vi "Lire Dividend.vi"(8 "error in (no error)":errorcluster caption="entrée d'erreur (pas d'erreur)", 11 "Share en entrée":refnum<class "Stock.lvclass">) -> (0 "error out":errorcluster caption="sortie d'erreur", 2 "Dividend":dbl, 3 "Share en sortie":refnum<class "Stock.lvclass">)   [LabVIEW 2012, in "Stock.lvclass"]
uses:
  Stock.lvclass
  Stock.lvclass/Stock.ctl
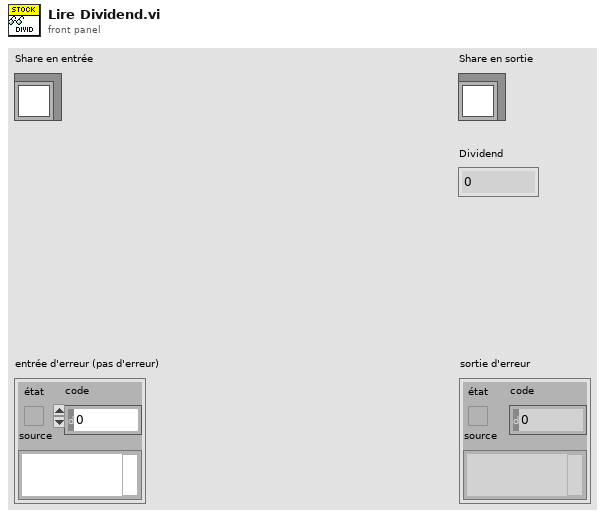
[diagram p1: front panel]
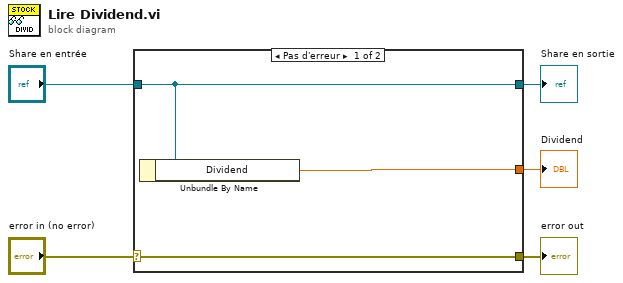
[diagram p0: block diagram]
diagram:
  n1 = case shown="Pas d'erreur" "error in (no error)" {
    selector: "error in (no error)" -> [w8 w9]
    tunnel: [w8 w9] -> w4
    tunnel: [w7 w10] -> w2
    tunnel: "Share en entrée" -> [w7 w10]
    tunnel: [w6 _] -> w1
    frame No Error {
      n2 = Unbundle By Name(w7) -> ("Dividend"=w6:dbl)
    }
    frame Error {
    }
  }
  "error out" <- w4
  "Share en sortie" <- w2
  "Dividend" <- w1
